vi "3.vi"(11 "文字列入力":string) -> (3 "文字列出力":string)   [LabVIEW 2019]
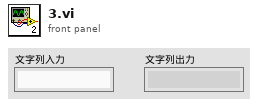
[diagram p1: front panel]
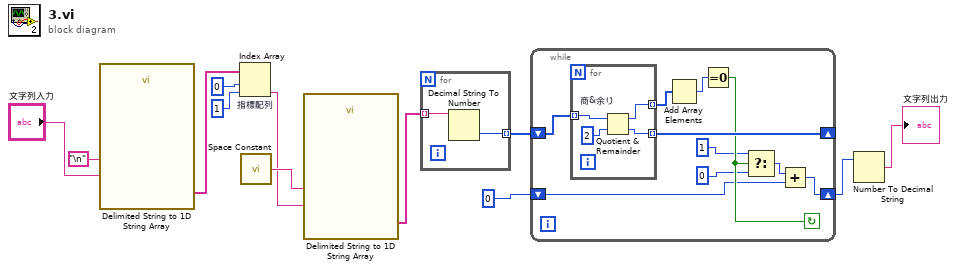
[diagram p0: block diagram]
diagram:
  n1 = call <vilib>:"Delimited String to 1D String Array.vi"("delimiter"="\n", "delimited string"="文字列入力") -> ("string array"=w5:string[])  [unwired: 9 in]
  n2 = Index Array "指標配列"(array=w5, index #1=0, index #2=1) -> (element #2=w6:string)  [unwired: 1 out]
  n3 = call <vilib>:"Space Constant.vi"() -> ("String"=w7:string)
  n4 = call <vilib>:"Delimited String to 1D String Array.vi"("delimiter"=w7, "delimited string"=w6) -> ("string array"=w8:string[])  [unwired: 9 in]
  n5 = for {
    tunnel: w8 -> [w14] mode=indexing
    tunnel: [w13] -> w9 mode=indexing
    n6 = Decimal String To Number(string=w14) -> (number=w13:i32)  [unwired: 2 in, 1 out]
  }
  n7 = while {
    shift-right: [w22] -> _
    shift-left: w9 -> [w24]
    shift-right: [w15] -> w11
    shift-left: 0 -> [w16]
    stop <- w20 continue-if-true
    n8 = for {
      tunnel: w24 -> [w28] mode=indexing
      tunnel: [w26] -> w22 mode=indexing
      tunnel: [w25] -> w23 mode=indexing
      n9 = Quotient & Remainder "商&余り"(x=w28, y=2) -> (x-y*floor(x/y)=w25:i32, floor(x/y)=w26:i32)
    }
    n10 = Add Array Elements(numeric array=w23) -> (sum=w21:i32)
    n11 = Equal To 0?(x=w21) -> (x = 0?=w20:bool)
    n12 = Select(t=1, s=w20, f=0) -> (s? t:f=w17:i32)
    n13 = Add(x=w17, y=w16) -> (x+y=w15:i32)
  }
  n14 = Number To Decimal String(number=w11) -> (decimal integer string=→"文字列出力":string)  [unwired: 1 in]
